vi "RSZVB Set Mixer Delay Upper Tone Source.vi"(7 "Port number (1)":i32=1, 8 "error in (no error)":errorcluster {"code" format="%.0x"}, 9 "Source (1)":i32(ring)=1 items=["None", "Port", "Generator"], 10 "Channel (1)":i32=1, 11 "VISA session":refnum<visa-resource-name>) -> (0 "error out":errorcluster {"code" format="%.0x"}, 3 "dup VISA session":refnum<visa-resource-name>)   [LabVIEW 2011]
doc: "Selects the source for the upper tone signal that is used for the mixer delay measurement.\n\nNotes:\n\n(1) This VI requires options R&S ZVA-K9 and R&S ZVA-K4.\n\nRemote-control command(s):\n[SENSe<Ch>:]FREQuency:MDELay:UTONe NONE | PORT | GENerator, <source_no>"
uses:
  _utility/RSZVB Global Data.vi
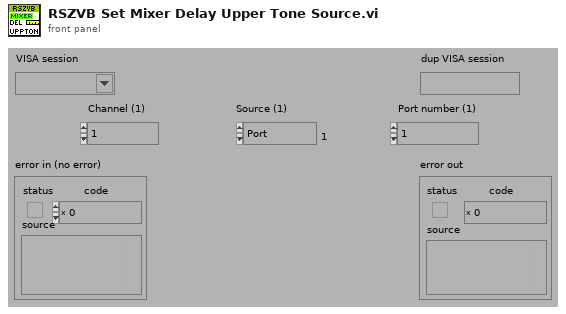
[diagram p1: front panel]
types:
  T1 = cluster{"Error Checking (T: On)":bool, "Installed Options":string[], "Data Valid?":bool, "Ports":i32, "Model":string[], "Option Checking (T: On)":bool}[]
  T2 = cluster{"Error Checking (T: On)":bool, "Installed Options":string[], "Data Valid?":bool, "Ports":i32, "Model":string[], "Option Checking (T: On)":bool}
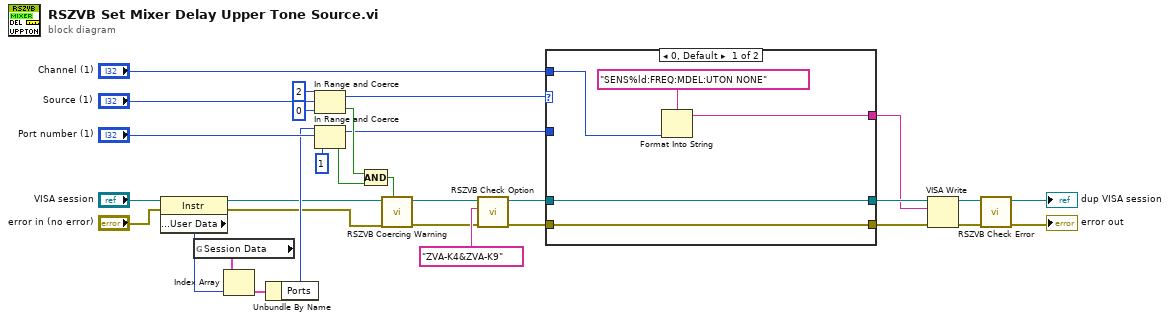
[diagram p0: block diagram]
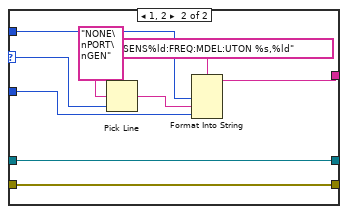
[diagram p2: hidden frame]
diagram:
  n1 = property class="Instr"(reference="VISA session", error in="error in (no error)") -> (reference out=w16:refnum<visa-resource-name>, error out=w17:errorcluster, "General Settings:User Data"=w29:u32)
  n2 = global read "RSZVB Global Data.vi" "Session Data"() -> (w30:T1)
  n3 = Index Array(array=w30, index=w29) -> (element=w31:T2)
  n4 = Unbundle By Name(w31) -> ("Ports"=w25:i32)
  n5 = In Range and Coerce(upper limit=2, x="Source (1)", lower limit=0) -> (coerced(x)=w12:i32, In Range?=w19:bool)
  n6 = In Range and Coerce(upper limit=w25, x="Port number (1)", lower limit=1) -> (coerced(x)=w8:i32, In Range?=w20:bool)
  n7 = Compound Arithmetic op=AND(w19, w20) -> (w18:bool)
  n8 = call "RSZVB Coercing Warning.vi"("In Range?"=w18, "error in (no error)"=w17, "VISA session"=w16) -> ("error out"=w13:errorcluster, "dup VISA session"=w14:refnum<visa-resource-name>)  [unwired: 7 in]
  n9 = call "RSZVB Check Option.vi"("error in (no error)"=w13, "Options"="ZVA-K4&ZVA-K9", "VISA session"=w14) -> ("error out"=w10:errorcluster, "dup VISA session"=w11:refnum<visa-resource-name>)  [unwired: 7 in]
  n10 = case shown="0, Default" w12 {
    selector: w12 -> [_ w42]
    tunnel: w11 -> [w36 w45]
    tunnel: w10 -> [w35 w44]
    tunnel: [w36 w45] -> w6
    tunnel: [w35 w44] -> w7
    tunnel: "Channel (1)" -> [w33 w40]
    tunnel: w8 -> [_ w38]
    tunnel: [w32 w37] -> w5
    frame 0, Default {
      n11 = Format Into String(format string="SENS%ld:FREQ:MDEL:UTON NONE", w33) -> (resulting string=w32:string)  [unwired: 2 in, 1 out]
    }
    frame 1, 2 {
      n12 = Pick Line(multi-line string="NONE\nPORT\nGEN", line index=w42) -> (output string=w39:string)  [unwired: 1 in]
      n13 = Format Into String(format string="SENS%ld:FREQ:MDEL:UTON %s,%ld", w40, w39, w38) -> (resulting string=w37:string)  [unwired: 2 in, 1 out]
    }
  }
  n14 = VISA Write(VISA resource name=w6, write buffer=w5, error in (no error)=w7) -> (VISA resource name out=w3:refnum<visa-resource-name>, error out=w4:errorcluster)  [unwired: 1 out]
  n15 = call "RSZVB Check Error.vi"("error in (no error)"=w4, "VISA session"=w3) -> ("error out"=→"error out":errorcluster, "dup VISA session"=→"dup VISA session":refnum<visa-resource-name>)  [unwired: 8 in]
